vi "PI_Num2Str.vi"(11 "x-Position":dbl) -> (3 "String":string)   [LabVIEW 2009]
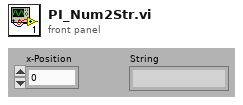
[diagram p1: front panel]
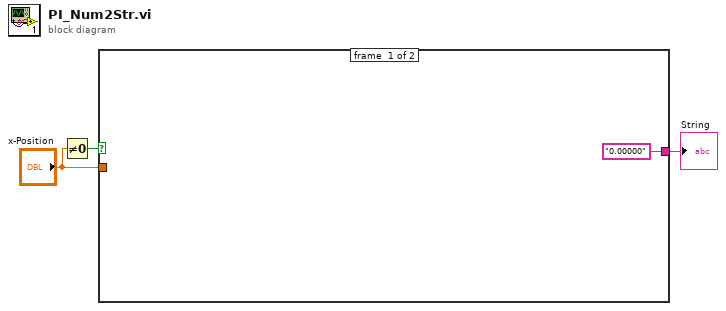
[diagram p0: block diagram]
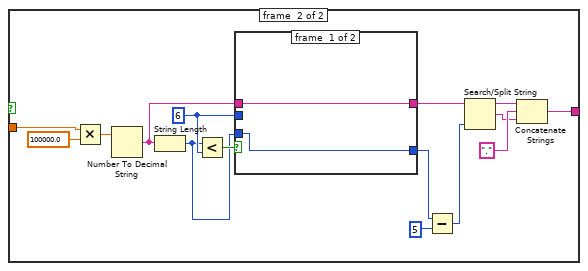
[diagram p2: hidden frame]
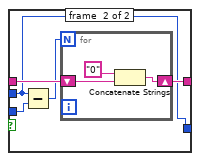
[diagram p3: hidden frame]
diagram:
  n1 = Not Equal To 0?(x="x-Position") -> (x != 0?=w1:bool)
  n2 = case shown="True" w1 {
    tunnel: ["0.00000" w19] -> w3
    tunnel: "x-Position" -> [_ w11]
    frame #0 {
    }
    frame #1 {
      w8 = 6 ("y")
      n3 = Multiply(x=w11, y=100000.0) -> (x*y=w12:dbl)
      n4 = Number To Decimal String(number=w12) -> (decimal integer string=w9:string)  [unwired: 1 out]
      n5 = String Length(string=w9) -> (length=w6:i32)
      n6 = Less?(x=w6, y=w8) -> (x < y?=w10:bool)
      n7 = case shown="False" w10 {
        tunnel: w9 -> [w21 w25]
        tunnel: w6 -> [w20 w24]
        tunnel: w8 -> [_ w22]
        tunnel: [w21 w26] -> w7
        tunnel: [w20 w22] -> w5
        frame #0 {
        }
        frame #1 {
          n8 = Subtract(x=w22, y=w24) -> (x-y=w23:i32)
          n9 = for {
            N: w23 -> [_]
            shift-right: [w28] -> w26
            shift-left: w25 -> [w27]
            n10 = Concatenate Strings("0", w27) -> (w28:string)
          }
        }
      }
      n11 = Subtract(x=w5, y=5) -> (x-y=w15:i32)
      n12 = Search/Split String(string=w7, offset (0)=w15) -> (substring before match=w16:string, match + rest of string=w17:string)  [unwired: 2 out]
      n13 = Concatenate Strings(w16, "." ("string"), w17) -> (w19:string)
    }
  }
  "String" <- w3
